vi "test Add Find Remove RAF CD.vi"(8 "error in (no error)":errorcluster, 11 "TestCase in":refnum<class "Switch Scripting Test Case.lvclass">) -> (0 "error out":errorcluster, 3 "TestCase out":refnum<class "Switch Scripting Test Case.lvclass">)   [LabVIEW 2017, in "Switch Scripting Test Case.lvclass"]
uses:
  Switch Scripting Test Case.lvclass
  C:/Program Files (x86)/National Instruments/LabVIEW 2017/vi.lib/addons/_JKI Toolkits/VI Tester/TestCase.llb/TestCase.lvclass
  <vilib>/addons/_JKI Toolkits/VI Tester/TestCase.llb/TestCase.lvclass
panel:
  in  "Save?":bool
  out "Output Filename":string
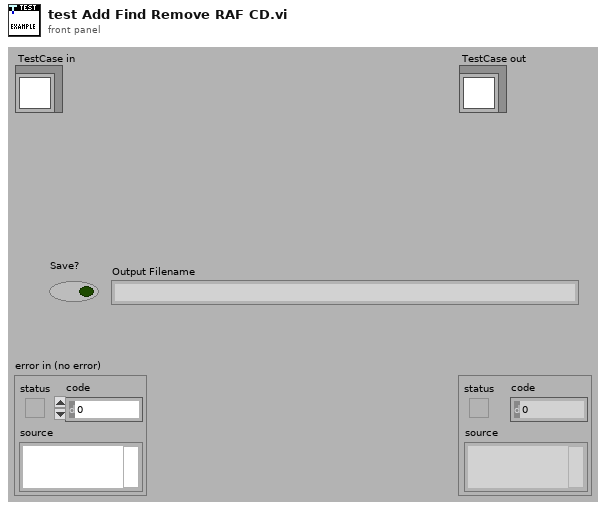
[diagram p1: front panel]
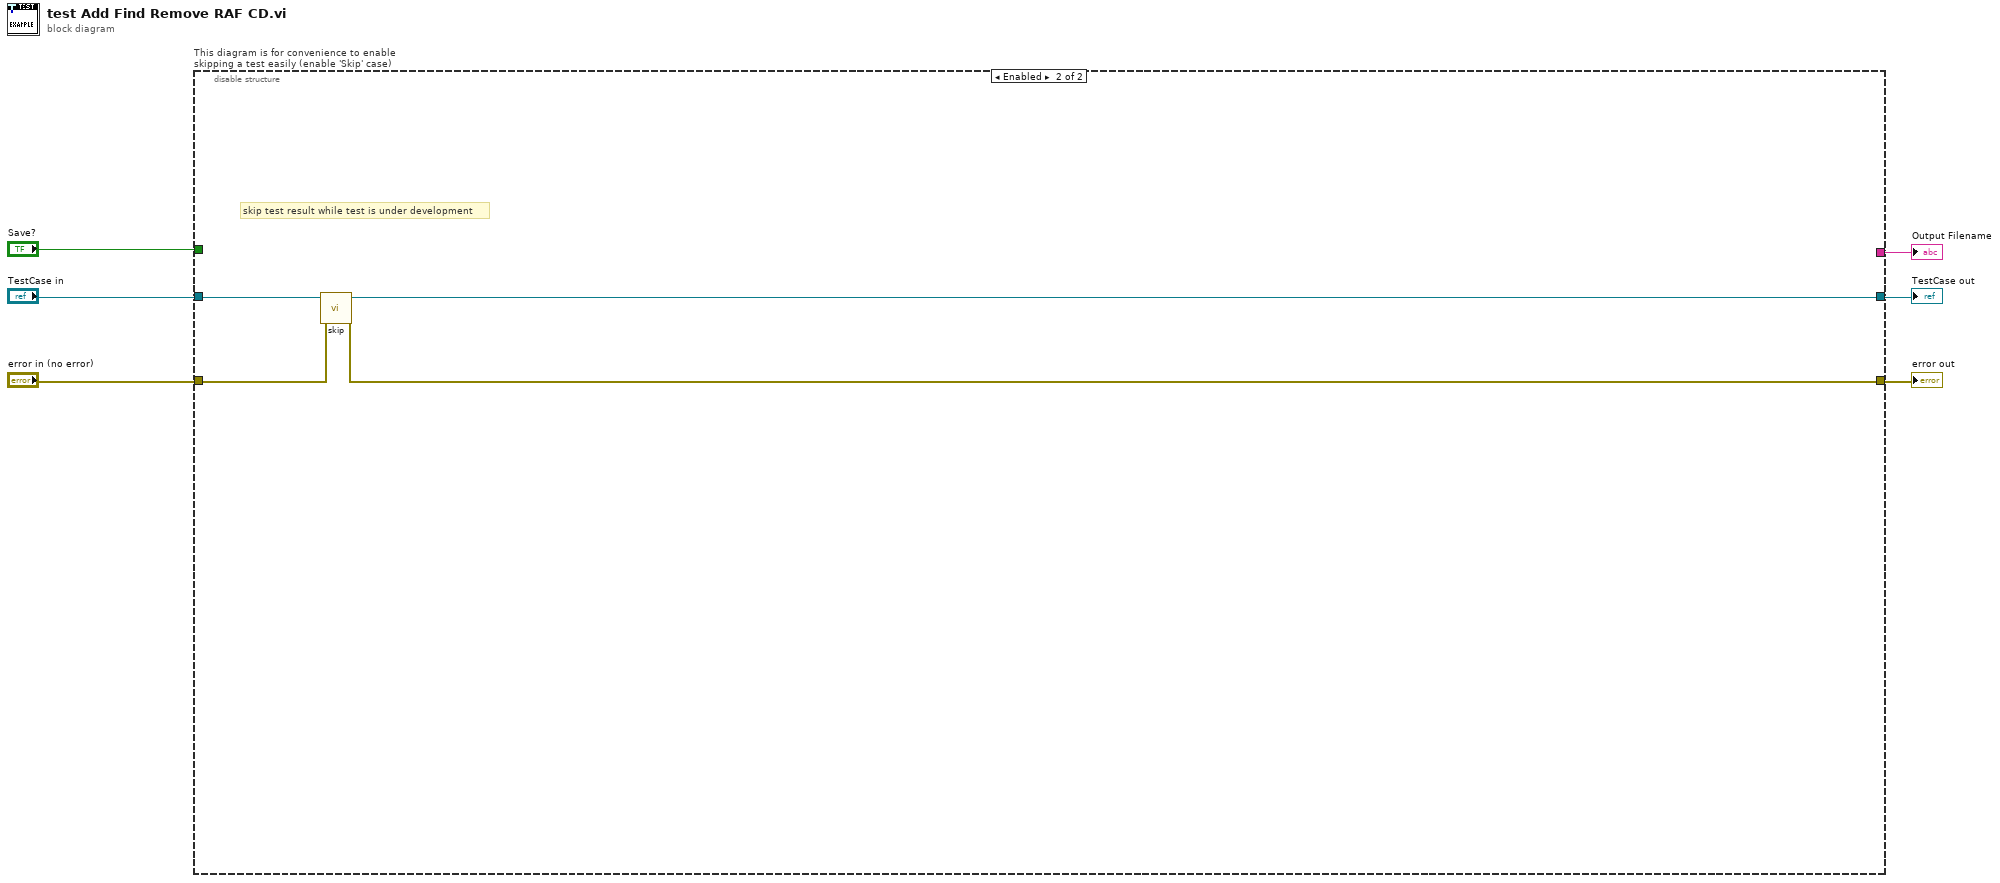
[diagram p0: block diagram]
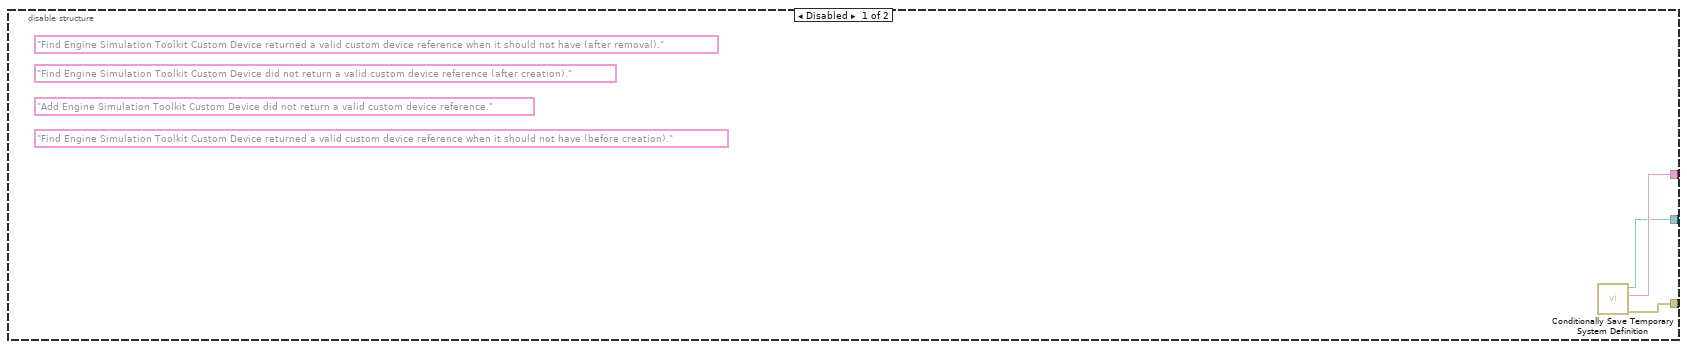
[diagram p2: hidden frame]
diagram:
  n1 = disable-structure "This diagram is for convenience to enable skipping a test easily (enable 'Skip' case)" shown="Enabled" {
    disable-tunnel: "TestCase in" -> [_ w13]
    disable-tunnel: [w7 w11] -> w3
    disable-tunnel: [w8 w12] -> w5
    disable-tunnel: "error in (no error)" -> [_ w10]
    disable-tunnel: [w9 _] -> w2
    disable-tunnel: "Save?" -> [_ _]
    frame Disabled {
      (unwired) "Find Engine Simulation Toolkit Custom Device returned a valid custom device reference when it should not have (after removal)." ("message (\"\")")
      (unwired) "Find Engine Simulation Toolkit Custom Device did not return a valid custom device reference (after creation)." ("message (\"\")")
      (unwired) "Find Engine Simulation Toolkit Custom Device returned a valid custom device reference when it should not have (before creation)." ("message (\"\")")
      (unwired) "Add Engine Simulation Toolkit Custom Device did not return a valid custom device reference." ("message (\"\")")
      n2 = call "Conditionally Save Temporary System Definition.vi"() -> ("error out"=w8:errorcluster, "filename"=w9:string, "Test Case"=w7:refnum<class "Switch Scripting Test Case.lvclass">)  [unwired: 9 in]
    }
    frame Enabled {
      # "skip test result while test is under development"
      n3 = call <vilib>:"skip.vi"("error in (no error)"=w10, "TestCase in"=w13) -> ("error out"=w12:errorcluster, "TestCase out"=w11:refnum<class "Switch Scripting Test Case.lvclass">)  [unwired: 8 in]
    }
  }
  "error out" <- w5
  "TestCase out" <- w3
  "Output Filename" <- w2
